vi "GSP_Manager_SCLNClient.vi"() -> ()   [LabVIEW 2015]
panel:
  in  "Config Path":path=path "C:/SOAR_Misc/GoodMan/Systems/Common/examples.cfg"
  out "Error In":errorcluster={"status"=TRUE, "code"=7, "source"="Open Config Data.vi"}
  out "Message Out":string
  out "Message In":string
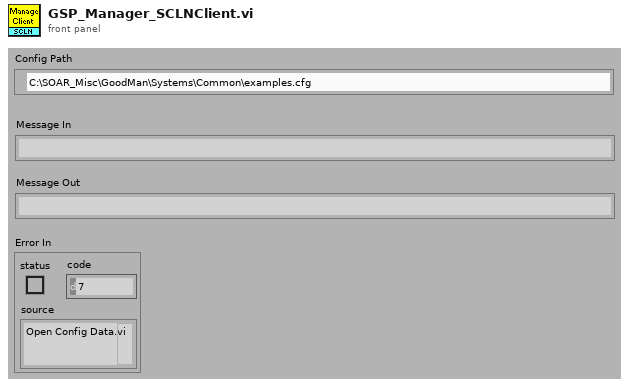
[diagram p1: front panel]
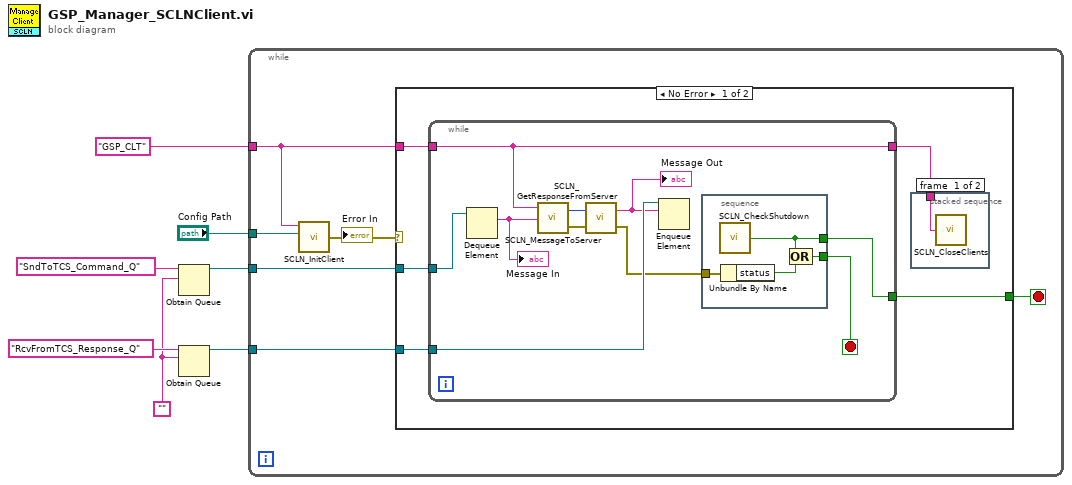
[diagram p0: block diagram]
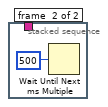
[diagram p2: hidden frame]
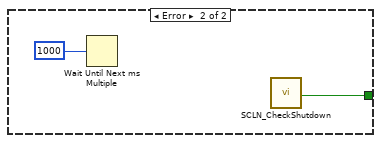
[diagram p3: hidden frame]
diagram:
  w3 = ""
  n1 = Obtain Queue(name (unnamed)="SndToTCS_Command_Q", element data type=w3) -> (queue out=w6:refnum<queue>)  [unwired: 3 in, 2 out]
  n2 = Obtain Queue(name (unnamed)="RcvFromTCS_Response_Q", element data type=w3) -> (queue out=w4:refnum<queue>)  [unwired: 3 in, 2 out]
  n3 = while {
    tunnel: w6 -> [w13]
    tunnel: w4 -> [w12]
    tunnel: "Config Path" -> [w11]
    tunnel: "GSP_CLT" ("String") -> [w10]
    stop <- w8 stop-if-true
    n4 = call "SCLN_InitClient.vi"("Config File Name"=w11, "Server Name"=w10) -> ("error out"=w9:errorcluster)  [unwired: 2 in]
    "Error In" <- w9
    n5 = case shown="No Error" w9 {
      tunnel: w13 -> [w18 _]
      tunnel: w12 -> [w17 _]
      tunnel: w10 -> [w16 _]
      tunnel: [w14 w36] -> w8
      frame No Error {
        n6 = while {
          tunnel: w18 -> [w28]
          tunnel: w17 -> [w27]
          tunnel: w16 -> [w22]
          tunnel: [w22] -> w15
          tunnel: [w21] -> w14
          stop <- w23 stop-if-true
          n7 = Dequeue Element(queue=w28) -> (element=w26:string)  [unwired: 2 in, 3 out]
          "Message In" <- w26
          n8 = call "SCLN_MessageToServer.vi"("Message"=w26, "Server Name"=w22) -> ("error out"=w30:errorcluster, "Index for Response"=w29:i32)  [unwired: 1 in]
          n9 = call "SCLN_GetResponseFromServer.vi"("error in (no error)"=w30, "Index for Response"=w29) -> ("error out"=w24:errorcluster, "Message"=w25:string)
          "Message Out" <- w25
          n10 = Enqueue Element(queue=w27, element=w25) -> ()  [unwired: 2 in, 3 out]
          n11 = stacked-sequence {
            tunnel: w24 -> [w34]
            tunnel: [w32] -> w23
            tunnel: [w31] -> w21
            frame #0 {
              n12 = call "SCLN_CheckShutdown.vi"() -> ("Shutdown"=w31:bool)
              n13 = Unbundle By Name(w34) -> ("status"=w33:bool)
              n14 = Compound Arithmetic op=OR(w31, w33) -> (w32:bool)
            }
          }
        }
        n15 = stacked-sequence {
          tunnel: w15 -> [w19 _]
          frame #0 {
            n16 = call "SCLN_CloseClients.vi"("Server Name"=w19) -> ()
          }
          frame #1 {
            n17 = Wait Until Next ms Multiple(millisecond multiple=500) -> ()  [unwired: 1 out]
          }
        }
      }
      frame Error {
        n18 = Wait Until Next ms Multiple(millisecond multiple=1000) -> ()  [unwired: 1 out]
        n19 = call "SCLN_CheckShutdown.vi"() -> ("Shutdown"=w36:bool)
      }
    }
  }
